vi "CloseVI.vi"(8 "error in":errorcluster, 11 "vi path":path) -> (0 "error out":errorcluster)   [LabVIEW 2011]
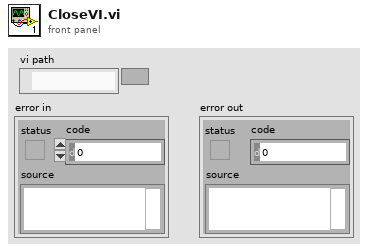
[diagram p1: front panel]
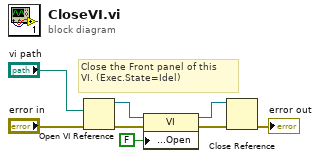
[diagram p0: block diagram]
diagram:
  # "Close the Front panel of this\nVI. (Exec.State=Idel)"
  n1 = Open VI Reference(vi path="vi path", error in (no error)="error in") -> (vi reference=w6:refnum<vi>, error out=w2:errorcluster)  [unwired: 4 in]
  n2 = property class="VI"(reference=w6, error in=w2, "Front Panel Window:Open"=FALSE) -> (reference out=w3:refnum<vi>, error out=w5:errorcluster)
  n3 = Close Reference(reference=w3, error in (no error)=w5) -> (error out=→"error out":errorcluster)
